vi "DriveNetwork.vi"(8 "error in (no error)":errorcluster) -> (0 "error out":errorcluster)   [LabVIEW 2023]
doc: "Network for Drive\n\nInputs:\n -- Error in -- Error cluster -- propagated error input\n\nOutputs:\n -- Error out -- Error cluster -- progated error output"
uses:
  DriveGlobal.vi
  <vilib>/Rock Robotics/Network Tables/NT Read Number.vi
  <vilib>/Rock Robotics/Network Tables/NT Write Number.vi
  <vilib>/Rock Robotics/Network Tables/NT Write Boolean.vi
  <vilib>/Rock Robotics/Network Tables/NT Read Boolean.vi
  <vilib>/Rock Robotics/WPI/ThirdParty/JAS_Junk/TrajLib/Trajectory_Library.lvlib
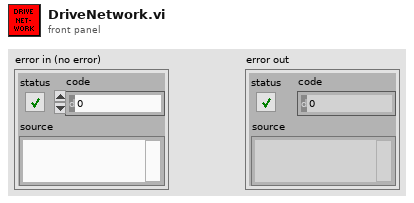
[diagram p1: front panel]
types:
  T1 = enum16{"Moving Average", "Low Pass 1st Order Butterworth", "Low Pass 2nd Order Butterworth", "High Pass 1st Order Butterworth", "High Pass 2nd Order Butterworth"}
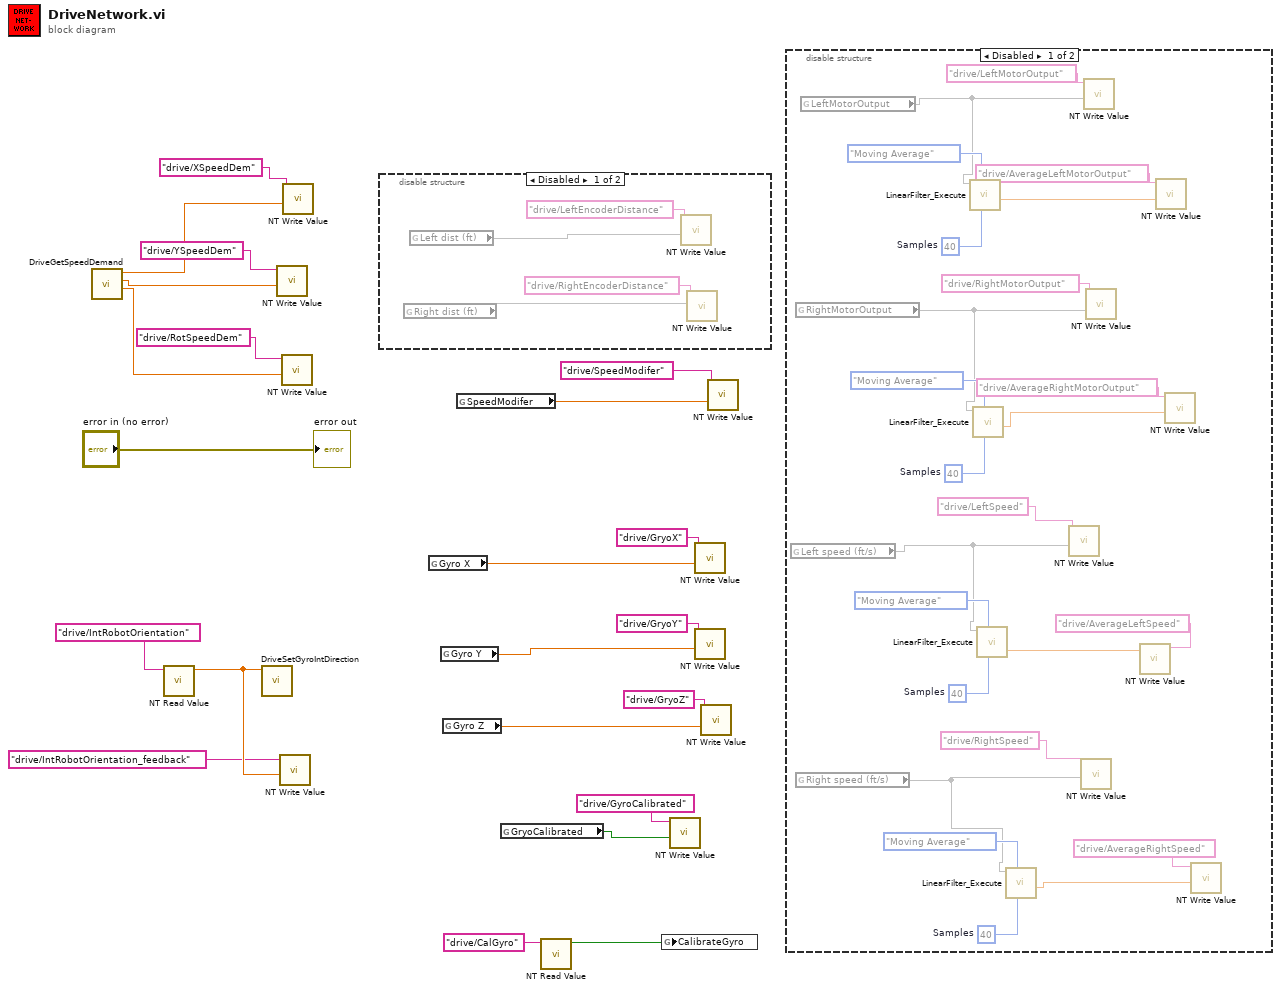
[diagram p0: block diagram]
diagram:
  n1 = call "DriveGetSpeedDemand.vi"() -> ("vOmega"=w4:dbl, "vY"=w20:dbl, "vX"=w21:dbl)  [unwired: 8 in, 1 out]
  n2 = call-poly <vilib>:"NT Read Value.vi"("name"="drive/IntRobotOrientation") -> ("value"=w2:dbl)  [unwired: 8 in, 2 out]
  n3 = call "DriveSetGyroIntDirection.vi"("GyroIntDirection"=w2) -> ()  [unwired: 11 in]
  n4 = call-poly <vilib>:"NT Write Value.vi"("value"=w20, "name"="drive/YSpeedDem") -> ()  [unwired: 9 in, 1 out]
  n5 = call-poly <vilib>:"NT Write Value.vi"("value"=w2, "name"="drive/IntRobotOrientation_feedback") -> ()  [unwired: 9 in, 1 out]
  n6 = call-poly <vilib>:"NT Write Value.vi"("value"=w4, "name"="drive/RotSpeedDem") -> ()  [unwired: 9 in, 1 out]
  n7 = call-poly <vilib>:"NT Write Value.vi"("value"=w21, "name"="drive/XSpeedDem") -> ()  [unwired: 9 in, 1 out]
  n8 = disable-structure shown="Disabled" {
    frame Disabled {
      n9 = global read "DriveGlobal.vi" "Right dist (ft)"() -> (w24)
      n10 = global read "DriveGlobal.vi" "Left dist (ft)"() -> (w23)
      n11 = call-poly <vilib>:"NT Write Value.vi"("value"=w23, "name"="drive/LeftEncoderDistance") -> ()  [unwired: 9 in, 1 out]
      n12 = call-poly <vilib>:"NT Write Value.vi"("value"=w24, "name"="drive/RightEncoderDistance") -> ()  [unwired: 9 in, 1 out]
    }
    frame Enabled {
    }
  }
  n13 = global read "DriveGlobal.vi" "Gyro X"() -> (w14:dbl)
  n14 = global read "DriveGlobal.vi" "Gyro Y"() -> (w15:dbl)
  n15 = global read "DriveGlobal.vi" "Gyro Z"() -> (w16:dbl)
  n16 = global read "DriveGlobal.vi" "SpeedModifer"() -> (w12:dbl)
  n17 = global read "DriveGlobal.vi" "GryoCalibrated"() -> (w6:bool)
  n18 = call-poly <vilib>:"NT Read Value.vi"("name"="drive/CalGyro") -> ("value"=w7:bool)  [unwired: 8 in, 2 out]
  n19 = global write "DriveGlobal.vi" "CalibrateGyro"(w7) -> ()
  n20 = call-poly <vilib>:"NT Write Value.vi"("value"=w6, "name"="drive/GyroCalibrated") -> ()  [unwired: 9 in, 1 out]
  n21 = call-poly <vilib>:"NT Write Value.vi"("value"=w14, "name"="drive/GryoX") -> ()  [unwired: 9 in, 1 out]
  n22 = call-poly <vilib>:"NT Write Value.vi"("value"=w15, "name"="drive/GryoY") -> ()  [unwired: 9 in, 1 out]
  n23 = call-poly <vilib>:"NT Write Value.vi"("value"=w16, "name"="drive/GryoZ") -> ()  [unwired: 9 in, 1 out]
  n24 = call-poly <vilib>:"NT Write Value.vi"("value"=w12, "name"="drive/SpeedModifer") -> ()  [unwired: 9 in, 1 out]
  n25 = disable-structure shown="Disabled" {
    frame Disabled {
      w42 = 40  # Samples
      w44 = 40  # Samples
      w46 = 40  # Samples
      w48 = 40  # Samples
      n26 = global read "DriveGlobal.vi" "Left speed (ft/s)"() -> (w35)
      n27 = global read "DriveGlobal.vi" "RightMotorOutput"() -> (w34)
      n28 = global read "DriveGlobal.vi" "Right speed (ft/s)"() -> (w36)
      n29 = global read "DriveGlobal.vi" "LeftMotorOutput"() -> (w33)
      n30 = call <vilib>:"LinearFilter_Execute.vi"("Samples"=w42, "Filter Type"=T1."Moving Average", "Input"=w33) -> ("Output"=w32:dbl)  [unwired: 7 in, 1 out]
      n31 = call <vilib>:"LinearFilter_Execute.vi"("Samples"=w44, "Filter Type"=T1."Moving Average", "Input"=w34) -> ("Output"=w31:dbl)  [unwired: 7 in, 1 out]
      n32 = call <vilib>:"LinearFilter_Execute.vi"("Samples"=w46, "Filter Type"=T1."Moving Average", "Input"=w35) -> ("Output"=w30:dbl)  [unwired: 7 in, 1 out]
      n33 = call <vilib>:"LinearFilter_Execute.vi"("Samples"=w48, "Filter Type"=T1."Moving Average", "Input"=w36) -> ("Output"=w29:dbl)  [unwired: 7 in, 1 out]
      n34 = call-poly <vilib>:"NT Write Value.vi"("value"=w35, "name"="drive/LeftSpeed") -> ()  [unwired: 9 in, 1 out]
      n35 = call-poly <vilib>:"NT Write Value.vi"("value"=w36, "name"="drive/RightSpeed") -> ()  [unwired: 9 in, 1 out]
      n36 = call-poly <vilib>:"NT Write Value.vi"("value"=w33, "name"="drive/LeftMotorOutput") -> ()  [unwired: 9 in, 1 out]
      n37 = call-poly <vilib>:"NT Write Value.vi"("value"=w34, "name"="drive/RightMotorOutput") -> ()  [unwired: 9 in, 1 out]
      n38 = call-poly <vilib>:"NT Write Value.vi"("value"=w30, "name"="drive/AverageLeftSpeed") -> ()  [unwired: 9 in, 1 out]
      n39 = call-poly <vilib>:"NT Write Value.vi"("value"=w32, "name"="drive/AverageLeftMotorOutput") -> ()  [unwired: 9 in, 1 out]
      n40 = call-poly <vilib>:"NT Write Value.vi"("value"=w31, "name"="drive/AverageRightMotorOutput") -> ()  [unwired: 9 in, 1 out]
      n41 = call-poly <vilib>:"NT Write Value.vi"("value"=w29, "name"="drive/AverageRightSpeed") -> ()  [unwired: 9 in, 1 out]
    }
    frame Enabled {
    }
  }
  "error out" <- "error in (no error)"
